vi "RSZVB Delete External Power Meter.vi"(8 "error in (no error)":errorcluster {"code" format="%.0x"}, 11 "VISA session":refnum<visa-resource-name>) -> (0 "error out":errorcluster {"code" format="%.0x"}, 3 "dup VISA session":refnum<visa-resource-name>)   [LabVIEW 2011]
doc: "This VI clears the configuration table for external power meters.\n\nRemote-control command(s):\nSYSTem:COMMunicate:RDEVice:PMETer<pmeter_no>:DELete"
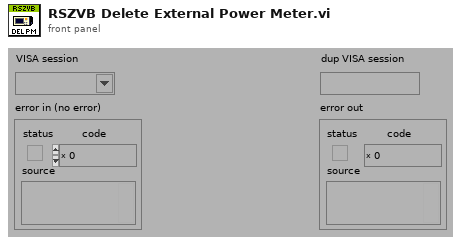
[diagram p1: front panel]
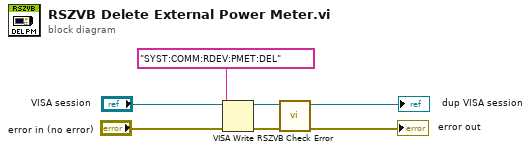
[diagram p0: block diagram]
diagram:
  n1 = VISA Write(VISA resource name="VISA session", write buffer="SYST:COMM:RDEV:PMET:DEL", error in (no error)="error in (no error)") -> (VISA resource name out=w6:refnum<visa-resource-name>, error out=w7:errorcluster)  [unwired: 1 out]
  n2 = call "RSZVB Check Error.vi"("error in (no error)"=w7, "VISA session"=w6) -> ("error out"=→"error out":errorcluster, "dup VISA session"=→"dup VISA session":refnum<visa-resource-name>)  [unwired: 8 in]
